vi "getLastDataPath.vi"(0 "文件夹输入":string="..\\CH1") -> (1 "数据文件名数组":string[](array[string]), 2 "文件夹路径":path)   [LabVIEW 2018]
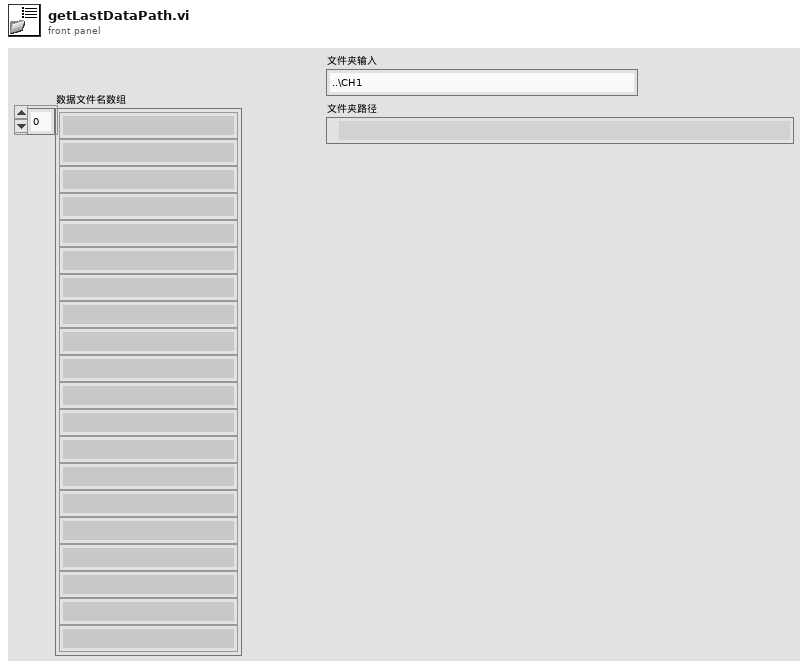
[diagram p1: front panel]
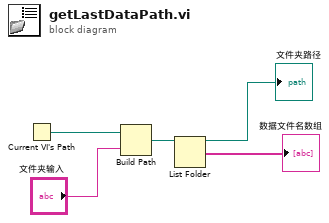
[diagram p0: block diagram]
diagram:
  n1 = Current VI's Path() -> (path=w5:path)
  n2 = Build Path(base path=w5, name or relative path="文件夹输入") -> (appended path=w4:path)
  n3 = List Folder(path=w4) -> (path out=→"文件夹路径":path, filenames=→"数据文件名数组":string[])  [unwired: 3 in, 2 out]
